vi "vhf_vehicle_dynamics.vi"(0 "Heading (Degrees)":dbl, 1 "Column":dbl, 2 "Vehicle Radius (meters)":dbl, 3 "Row":dbl, 4 "Robot Pos (Squares)":cluster{dbl, dbl}, 5 "Grid Resolution (meters)":dbl, 7 "Turning Radius (meters)":dbl) -> (6 "No Right":bool, 8 "No Left":bool)   [LabVIEW 2010]
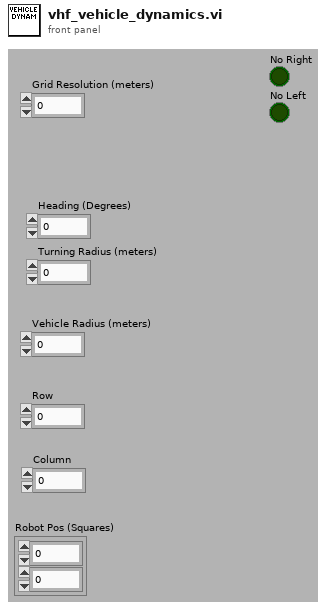
[diagram p1: front panel]
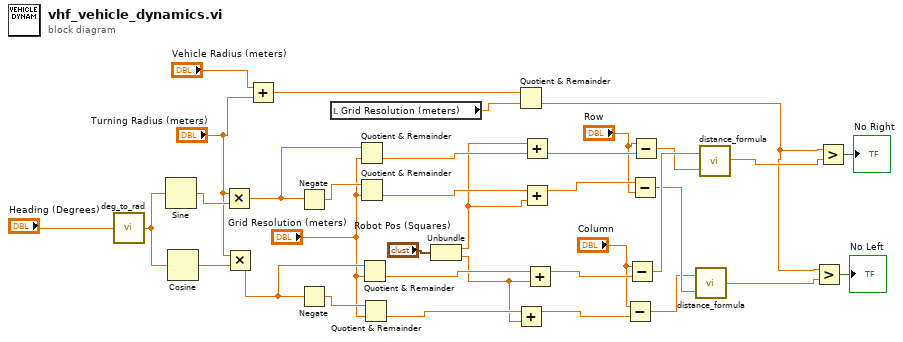
[diagram p0: block diagram]
diagram:
  n1 = call "deg_to_rad.vi"("Degrees"="Heading (Degrees)") -> ("Radians"=w34:dbl)
  n2 = Sine(x=w34) -> (sin(x)=w32:dbl)
  n3 = Cosine(x=w34) -> (cos(x)=w33:dbl)
  n4 = Multiply(x="Turning Radius (meters)", y=w32) -> (x*y=w31:dbl)
  n5 = Multiply(x="Turning Radius (meters)", y=w33) -> (x*y=w29:dbl)
  n6 = Add(x="Vehicle Radius (meters)", y="Turning Radius (meters)") -> (x+y=w7:dbl)
  n7 = Negate(x=w31) -> (-x=w30:dbl)
  n8 = Negate(x=w29) -> (-x=w28:dbl)
  n9 = local read "Grid Resolution (meters)"() -> (w4:dbl)
  n10 = Quotient & Remainder(x=w31, y="Grid Resolution (meters)") -> (floor(x/y)=w26:dbl)  [unwired: 1 out]
  n11 = Quotient & Remainder(x=w30, y="Grid Resolution (meters)") -> (floor(x/y)=w25:dbl)  [unwired: 1 out]
  n12 = Quotient & Remainder(x=w29, y="Grid Resolution (meters)") -> (floor(x/y)=w24:dbl)  [unwired: 1 out]
  n13 = Quotient & Remainder(x=w28, y="Grid Resolution (meters)") -> (floor(x/y)=w23:dbl)  [unwired: 1 out]
  n14 = Unbundle("Robot Pos (Squares)") -> (w9:dbl, w8:dbl)
  n15 = Quotient & Remainder(x=w7, y=w4) -> (floor(x/y)=w3:dbl)  [unwired: 1 out]
  n16 = Add(x=w23, y=w8) -> (x+y=w12:dbl)
  n17 = Add(x=w9, y=w26) -> (x+y=w10:dbl)
  n18 = Add(x=w25, y=w9) -> (x+y=w11:dbl)
  n19 = Add(x=w24, y=w8) -> (x+y=w13:dbl)
  n20 = Subtract(x="Column", y=w12) -> (x-y=w19:dbl)
  n21 = Subtract(x="Column", y=w13) -> (x-y=w22:dbl)
  n22 = Subtract(x=w11, y="Row") -> (x-y=w20:dbl)
  n23 = Subtract(x="Row", y=w10) -> (x-y=w21:dbl)
  n24 = call "distance_formula.vi"("X2 - X1"=w20, "Y2 - Y1"=w19) -> ("Distance"=w6:dbl)
  n25 = call "distance_formula.vi"("X2 - X1"=w21, "Y2 - Y1"=w22) -> ("Distance"=w5:dbl)
  n26 = Greater?(x=w3, y=w6) -> (0:→"No Left":bool)
  n27 = Greater?(x=w3, y=w5) -> (0:→"No Right":bool)
